vi "Move To Pos.vi"(0 "Lifter_motor in":refnum<class "Lifter_motor.lvclass">, 1 "Step In range":bool, 5 "Step Distance":dbl, 7 "ADC distance":dbl, 9 "Possition selector":T1(radio), 11 "error in (no error)":errorcluster) -> (4 "Lifter_motor out":refnum<class "Lifter_motor.lvclass">, 6 "Driver ACK?":bool, 15 "error out":errorcluster)   [LabVIEW 2019, in "Lifter_motor.lvclass"]
uses:
  Lifter_motor.lvclass
  Lifter_motor.lvclass/Lifter_motor.ctl
  TCP Class/LifterTCP.lvclass
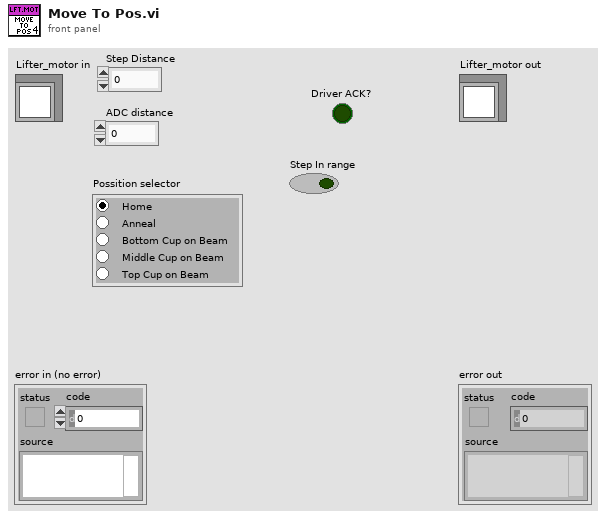
[diagram p1: front panel]
types:
  T1 = enum32{"Home", "Anneal", "Bottom Cup on Beam", "Middle Cup on Beam", "Top Cup on Beam"}
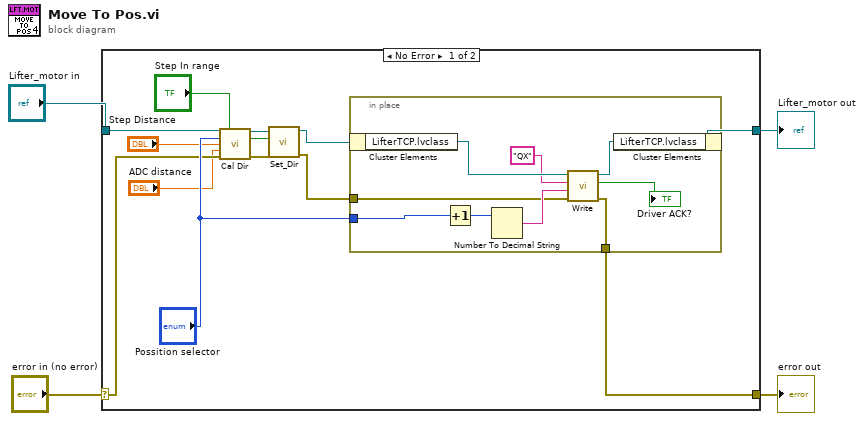
[diagram p0: block diagram]
diagram:
  n1 = case shown="No Error" "error in (no error)" {
    selector: "error in (no error)" -> [w9 w28]
    tunnel: [w11 w28] -> w3
    tunnel: [w17 w27] -> w1
    tunnel: "Lifter_motor in" -> [w16 w27]
    frame No Error {
      n2 = call "Cal Dir.vi"("Lifter_motor in"=w16, "Step In range"="Step In range", "Possition selector"="Possition selector", "Step Count"="Step Distance", "ADC distance"="ADC distance", "error in (no error)"=w9) -> ("Lifter_motor out"=w14:refnum<class "Lifter_motor.lvclass">, "Direction"=w13:bool, "error out"=w10:errorcluster)  [unwired: 7 in]
      n3 = call "Set_Dir.vi"("error in (no error)"=w10, "Direction"=w13, "Lifter_motor in"=w14) -> ("error out"=w8:errorcluster, "Lifter_motor out"=w12:refnum<class "Lifter_motor.lvclass">)  [unwired: 6 in, 1 out]
      n4 = in-place {
        in-place-border: "Possition selector" -> [w20]
        in-place-border: [w19] -> w11
        in-place-border: w8 -> [w18]
        n5 = in-place-cluster #1(w12) -> ("LifterTCP.lvclass"=w26:refnum<class "LifterTCP.lvclass">)
        n6 = Increment(x=w20) -> (x+1=w24:u32)
        n7 = Number To Decimal String(number=w24) -> (decimal integer string=w22:string)  [unwired: 1 in]
        n8 = call "Write.vi"("error in (no error)"=w18, "Parameter 2"=w22, "Parameter 1"="QX" ("string"), "LifterTCP in"=w26) -> ("error out"=w19:errorcluster, "Driver ACK?"=→"Driver ACK?":bool, "LifterTCP out"=w25:refnum<class "LifterTCP.lvclass">)  [unwired: 5 in]
        n9 = in-place-cluster #1("LifterTCP.lvclass"=w25) -> (w17:refnum<class "Lifter_motor.lvclass">)
      }
    }
    frame Error {
    }
  }
  "error out" <- w3
  "Lifter_motor out" <- w1
